vi "Configure Posts Binding.vi"(8 "error in (no error)":errorcluster, 10 "Output Post Binding (0: AUX)":i32(ring) items=["AUX", "20A"], 11 "VISA resource name":refnum<visa-resource-name>) -> (0 "error out":errorcluster, 3 "VISA resource name out":refnum<visa-resource-name>)   [LabVIEW 2012, in "Fluke 5080.lvlib"]
doc: "Selects the active binding posts for current output. \n\nNote:\n(1) This applies to current and power outputs.\n(2) The current post setting is retained until the power is turned off or the Rest button is pressed."
uses:
  <instrlib>/Fluke 5080/Fluke 5080.lvlib
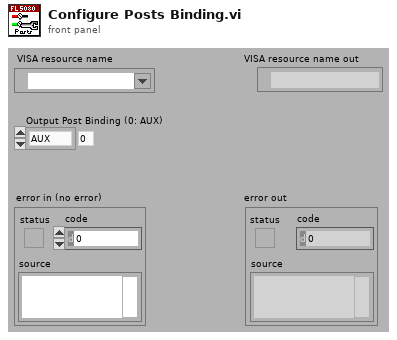
[diagram p1: front panel]
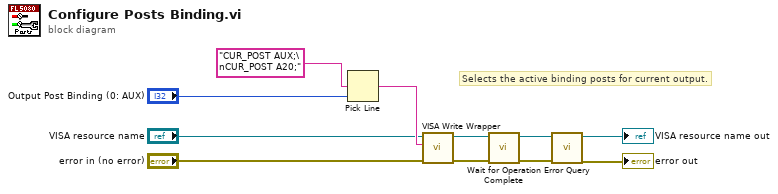
[diagram p0: block diagram]
diagram:
  # "Selects the active binding posts for current output."
  n1 = Pick Line(multi-line string="CUR_POST AUX;\nCUR_POST A20;", line index="Output Post Binding (0: AUX)") -> (output string=w9:string)  [unwired: 1 out]
  n2 = call <instrlib>:"VISA Write Wrapper.vi"("error in (no error)"="error in (no error)", "Write Buffer"=w9, "VISA resource name"="VISA resource name") -> ("error out"=w1:errorcluster, "VISA resource name out"=w2:refnum<visa-resource-name>)  [unwired: 7 out]
  n3 = call <instrlib>:"Wait for Operation Complete.vi"("error in (no error)"=w1, "VISA resource name"=w2) -> ("error out"=w3:errorcluster, "VISA resource name out"=w4:refnum<visa-resource-name>)  [unwired: 8 in]
  n4 = call <instrlib>:"Error Query.vi"("error in (no error)"=w3, "VISA resource name"=w4) -> ("error out"=→"error out":errorcluster, "VISA resource name out"=→"VISA resource name out":refnum<visa-resource-name>)  [unwired: 8 out]
